vi "Path2Obs.vi"() -> (0 "Path":path)   [LabVIEW 2019]
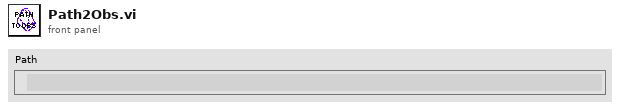
[diagram p1: front panel]
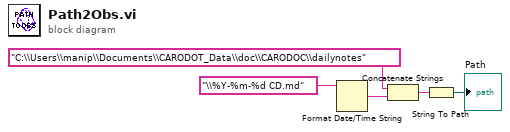
[diagram p0: block diagram]
diagram:
  n1 = Format Date/Time String(time format string (%c)="\\%Y-%m-%d CD.md") -> (date/time string=w5:string)  [unwired: 2 in]
  n2 = Concatenate Strings("C:\\Users\\manip\\Documents\\CARODOT_Data\\doc\\CARODOC\\dailynotes", w5) -> (w2:string)
  n3 = String To Path(string=w2) -> (path=→"Path":path)
